vi "PressureSensor.vi"(7 "Enum":T4, 8 "error in (no error)":errorcluster, 10 "PressureScaler":dbl, 11 "AIDeviceRef 3":T1={"DevStatus"={"status"=FALSE, "code"=0, "source"=""}, "Analog Module"=enum."Analog Module 1", "Analog Channel"=enum."Invalid"}) -> (0 "error out":errorcluster, 3 "Pressure":dbl)   [LabVIEW 2013]
uses:
  PressureSensorMode.ctl
  <vilib>/Rock Robotics/WPI/AnalogChannel/WPI_AnalogChannelDevRef.ctl
  <vilib>/Rock Robotics/SystemInterfaces/Typedef/FPGA_TypedefAnalogModule.ctl
  <vilib>/Rock Robotics/SystemInterfaces/AI/FPGA_AIChannel.ctl
panel:
  in  "Samples Per Second":dbl
  in  "AverageBits":u8
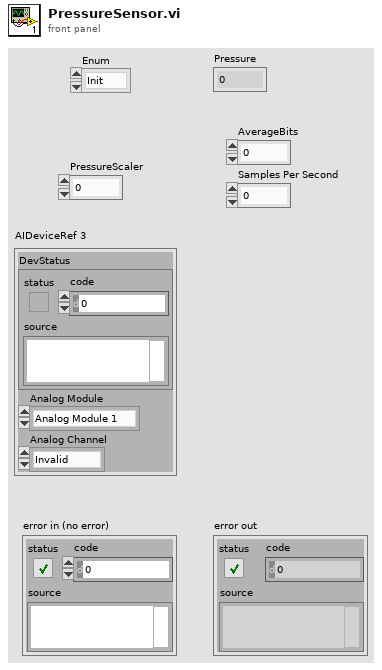
[diagram p1: front panel]
types:
  T1 = typedef "WPI_AnalogChannelDevRef.ctl" = cluster{"DevStatus":errorcluster, "Analog Module":T2, "Analog Channel":T3}
  T2 = typedef "FPGA_TypedefAnalogModule.ctl" = enum16{"Analog Module 1", "Analog Module 2"}
  T3 = typedef "FPGA_AIChannel.ctl" = enum8{"AI 1", "AI 2", "AI 3", "AI 4", "AI 5", "AI 6", "AI 7", "AI 8", "Invalid"}
  T4 = typedef "PressureSensorMode.ctl" = enum16{"Init", "ReadValue", "Disable"}
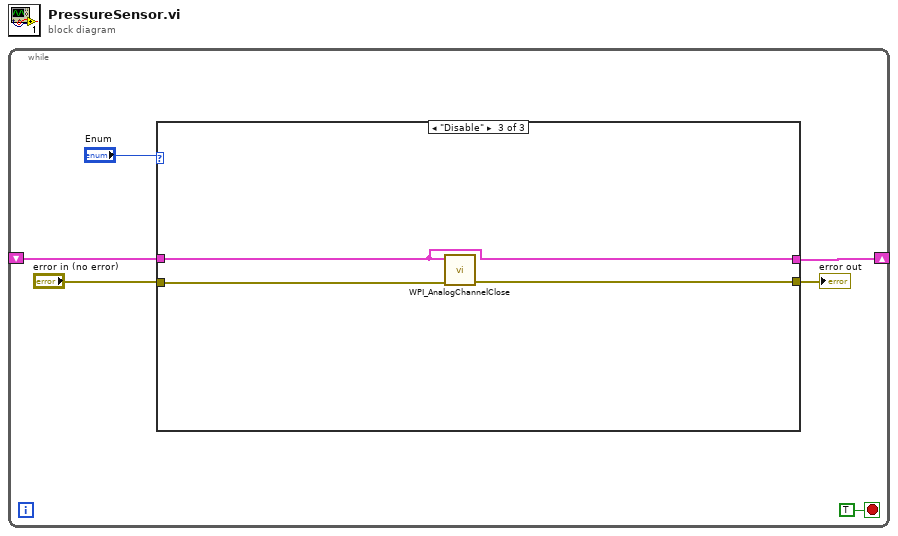
[diagram p0: block diagram]
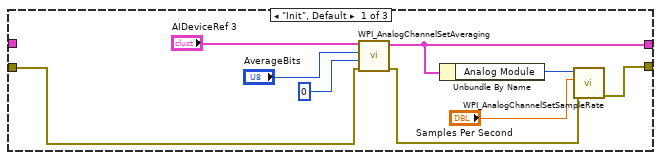
[diagram p2: hidden frame]
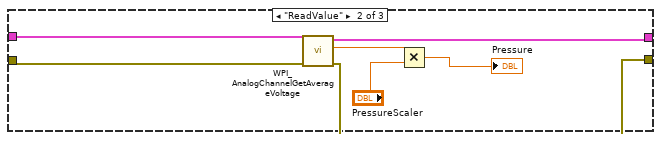
[diagram p3: hidden frame]
diagram:
  n1 = while {
    shift-right: [w5] -> _
    shift-left: _ -> [w4]
    stop <- TRUE stop-if-true
    n2 = case shown="\"Disable\"" "Enum" {
      tunnel: [w14 w21 w23] -> w5
      tunnel: w4 -> [_ w22 w23]
      tunnel: "error in (no error)" -> [w9 w17 w25]
      tunnel: [w7 w16 w24] -> w2
      frame "Init", Default {
        n3 = call <vilib>:"WPI_AnalogChannelSetAveraging.vi"("error in (no error)"=w9, "OversampleBits"=u8 0, "AverageBits"="AverageBits", "AIDeviceRef"="AIDeviceRef 3") -> ("error out"=w8:errorcluster, "AIDeviceRef"=w14:T1)  [unwired: 6 out]
        n4 = Unbundle By Name(w14) -> ("Analog Module"=w13:T2)
        n5 = call <vilib>:"WPI_AnalogChannelSetSampleRate.vi"("error in (no error)"=w8, "Samples Per Second"="Samples Per Second", "Analog Module (Module 1)"=w13) -> ("error out"=w7:errorcluster)  [unwired: 1 in, 7 out]
      }
      frame "ReadValue" {
        n6 = call <vilib>:"WPI_AnalogChannelGetAverageVoltage.vi"("error in (no error)"=w17, "AIDeviceRef"=w22) -> ("error out"=w16:errorcluster, "Voltage"=w20:dbl, "AIDeviceRef"=w21:T1)  [unwired: 7 out]
        n7 = Multiply(x=w20, y="PressureScaler") -> (x*y=→"Pressure":dbl)
      }
      frame "Disable" {
        n8 = call <vilib>:"WPI_AnalogChannelClose.vi"("error in (no error)"=w25, "AIDeviceRef"=w23) -> ("error out"=w24:errorcluster)  [unwired: 9 in]
      }
    }
    "error out" <- w2
  }
